vi "PNG Loader Tool.vi"() -> ()   [LabVIEW 2020, in "PicoG-Core.lvlib"]
uses:
  PicoG-Core.lvlib
panel:
  out "error out":errorcluster
  in  "Path":path=path "Z:/shared/picog/boards/chip.png"
  out "new picture":picture
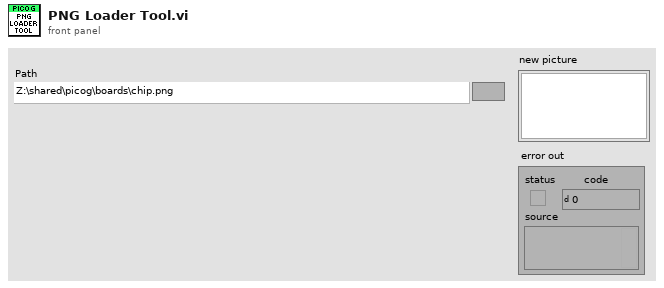
[diagram p1: front panel]
types:
  T1 = typedef "imagedata.ctl" = cluster{"image type":i32, "image depth":i32, "image":u8[], "mask":u8[], "colors":u32[], "Rectangle":cluster{"left":i16, "top":i16, "right":i16, "bottom":i16}}
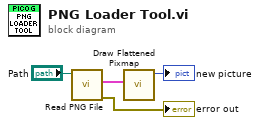
[diagram p0: block diagram]
diagram:
  n1 = call <vilib>:"Read PNG File.vi"("path to PNG file"="Path") -> ("error out"=→"error out":errorcluster, "image data"=w3:T1)  [unwired: 8 in, 1 out]
  n2 = call <vilib>:"Draw Flattened Pixmap.vi"("image data"=w3) -> ("new picture"=→"new picture":picture)  [unwired: 8 in]
